vi "wf_amp_multi.vi"(8 "error in":errorcluster, 10 "value":dbl=0.1) -> (0 "error out":errorcluster, 2 "value out":dbl=-3.829999999999993)   [LabVIEW 2017]
panel:
  in  "Devices":T1(array[cluster])=[{"device"="WFG_A", "channel"=1, "scale"=1.0}] {"scale" min=0.01 max=100.0; "channel" items=["1"=1, "2"=2]}
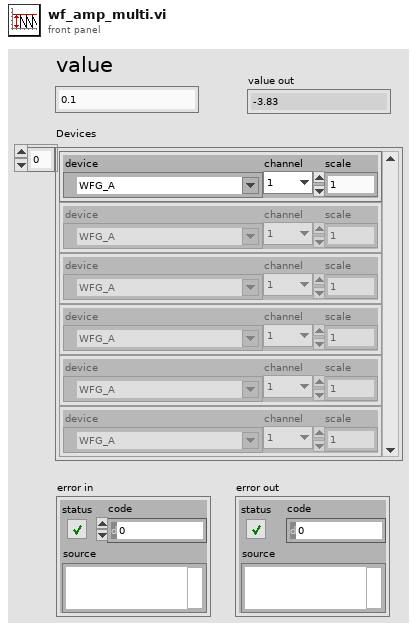
[diagram p1: front panel]
types:
  T1 = cluster{"device":refnum<visa-resource-name>, "channel":u8, "scale":dbl}[]
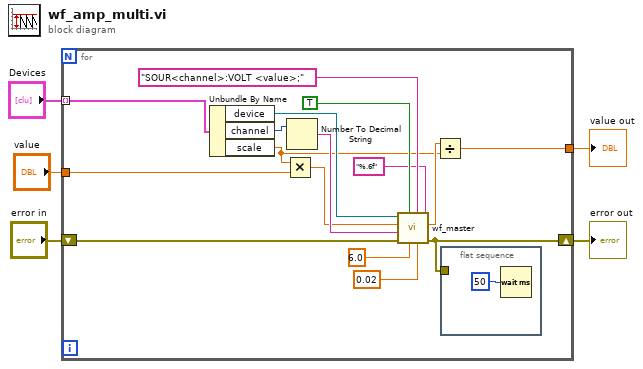
[diagram p0: block diagram]
diagram:
  n1 = for {
    tunnel: "Devices" -> [w18] mode=indexing
    shift-right: [w11] -> w3
    shift-left: "error in" -> [w19]
    tunnel: [w6] -> w2
    tunnel: "value" -> [w10]
    n2 = Unbundle By Name(w18) -> ("device"=w17:refnum<visa-resource-name>, "channel"=w13:u8, "scale"=w7:dbl)
    n3 = Multiply(x=w7, y=w10) -> (x*y=w9:dbl)
    n4 = Number To Decimal String(number=w13) -> (decimal integer string=w12:string)  [unwired: 1 in]
    n5 = call "wf_master.vi"("format"="%.6f", "lower limit"=0.02, "template"="SOUR<channel>:VOLT <value>;", "upper limit"=6.0, "override"=TRUE, "error in (no error)"=w19, "options"=w12, "value"=w9, "VISA IN"=w17) -> ("error out"=w11:errorcluster, "value out"=w8:dbl)  [unwired: 1 in]
    n6 = Divide(x=w8, y=w7) -> (x/y=w6:dbl)
    n7 = flat-sequence {
      tunnel: w11 -> [_]
      frame #0 {
        n8 = Wait (ms)(milliseconds to wait=u32 50) -> ()  [unwired: 1 out]
      }
    }
  }
  "error out" <- w3
  "value out" <- w2
